vi "FGPA_HoppingStep(Nonlinear-ZOnly).vi"() -> ()   [LabVIEW 2014]
uses:
  <vilib>/Platform/TimedLoop/XDataNode/timing_clust.ctl
  <vilib>/Platform/TimedLoop/XDataNode/nitl_modes.ctl
  <vilib>/Platform/TimedLoop/XDataNode/wakeup.ctl
  <vilib>/rvi/Emulation/niFpgaSctlEmulationGetInTimedLoop.vi
  <vilib>/rvi/eio/common/nirviEmuTemplateMethod_errors.vi
  <vilib>/rvi/Emulation/niFpgaGetClockAttributes.vi
  <vilib>/rvi/Emulation/niFpgaEmulationReportErrorSimple.vi
  <vilib>/rvi/Emulation/niFpgaProcessEmulError.vi
  <vilib>/rvi/Emulation/niFpgaCriticalErrorInLSC.vi
  <vilib>/rvi/interface/RandomDataEmulation/niFpgaRandomDataHandleErrors.vi
  <vilib>/eio/EIONode/EIONode.xnode
  <vilib>/Platform/TimedLoop/XDataNode/XDataNode.xnode
  <vilib>/rvi/DataTransferAndStorage/Container/XNode/niFpgaContainer.xnode
  <vilib>/rvi/interface/RandomDataEmulation/nirviRandomDataFpgaReadWriteTemplate.vi
  <vilib>/Platform/TimedLoop/XDataNode/XDNodeRunTimeDep.lvlib
panel:
  in  "Relative?":bool
  in  "RelativeWithdraw":i16
  in  "BottomSleep us":i16=120
  in  "UpperSleep us":i16=120
  out "ZRealPos":i16
  out "Waveform Chart":i32(graph)
  in  "stop":bool
  out "Z":i32(graph)
  in  "ZOffset":i16
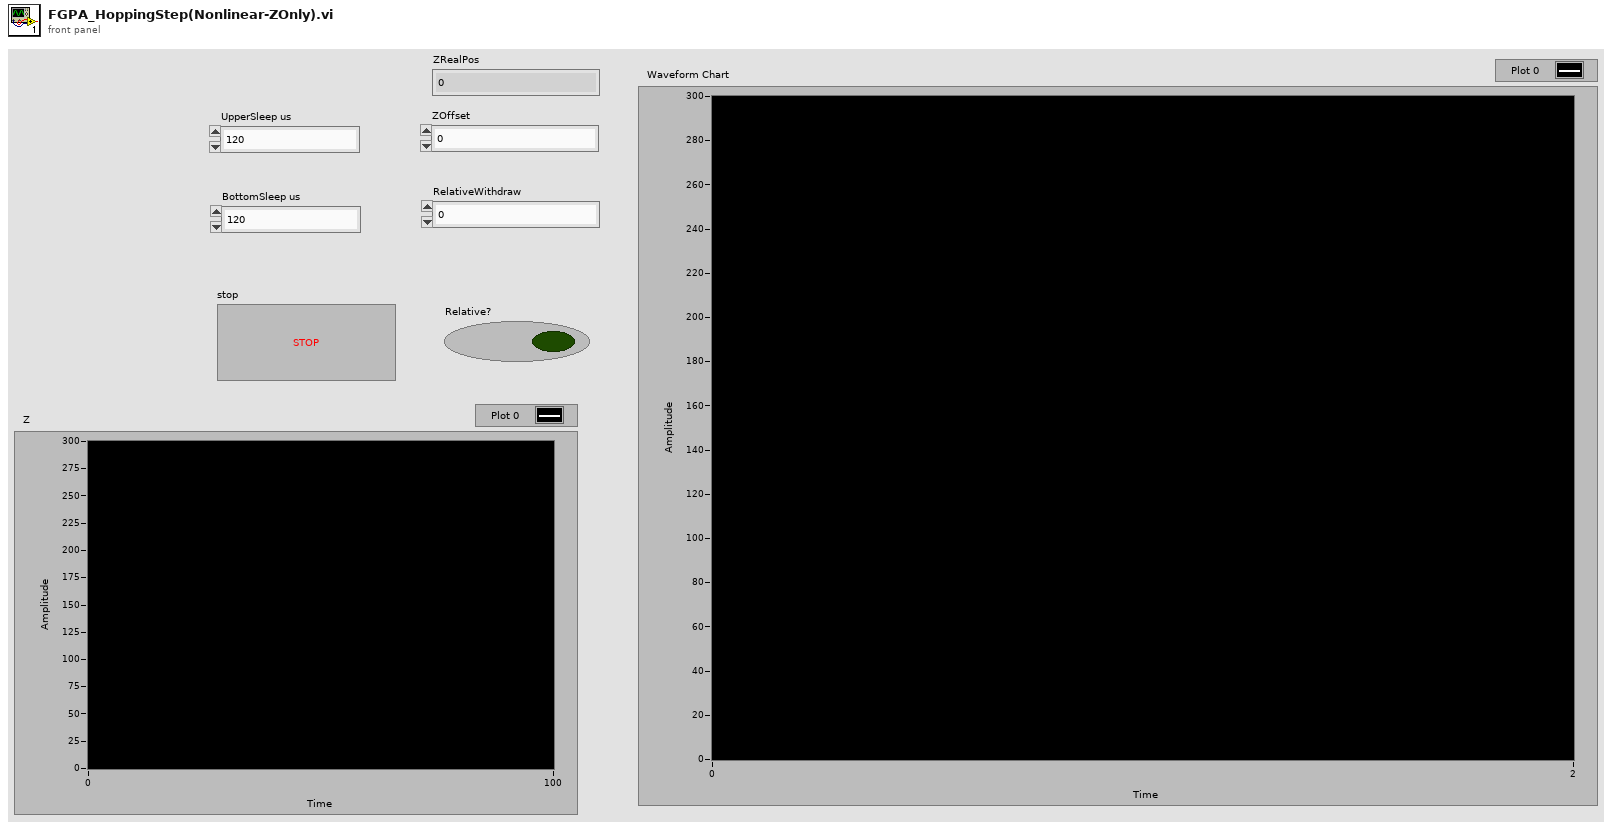
[diagram p1: front panel]
types:
  T1 = typedef "XDNodeRunTimeDep.lvlib/timing_clust.ctl" = cluster{"Expected End [f-1]":u64, "Actual End [f-1]":u64, "Finished Late? [f-1]":bool, "Expected End [i-1]":u64, "Actual End [i-1]":u64, "Finished Late? [i-1]":bool, "Expected Start [i]":u64, "Actual Start [i]":u64, "Expected Start [f]":u64, "Actual Start [f]":u64, "Source Name":string, "Structure Name":string, "Period":i64, "Deadline":i64, "Offset":i64, "Start":i64, "Priority":i32, "Timeout":i32, "Mode":T2, "Wakeup Reason":T3, "Error":errorcluster, "Source Type":string, "Secondary Source Type":string, "Global End Time":u64, "Global Start Time":u64, "Frame Duration":u64, "Iteration Duration":u64, "Assigned CPU":i32, "I/O Scan Engine Mode":u32}
  T2 = typedef "XDNodeRunTimeDep.lvlib/nitl_modes.ctl" = enum32{"No Change", "Process missed periods, maintain original phase", "Discard missed periods, maintain original phase", "Process missed periods, ignore original phase", "Discard missed periods, ignore original phase"}
  T3 = typedef "XDNodeRunTimeDep.lvlib/wakeup.ctl" = enum32{"Normal", "Aborted", "Asynchronous wakeup", "Timing source error", "Timed loop error", "Timeout"}
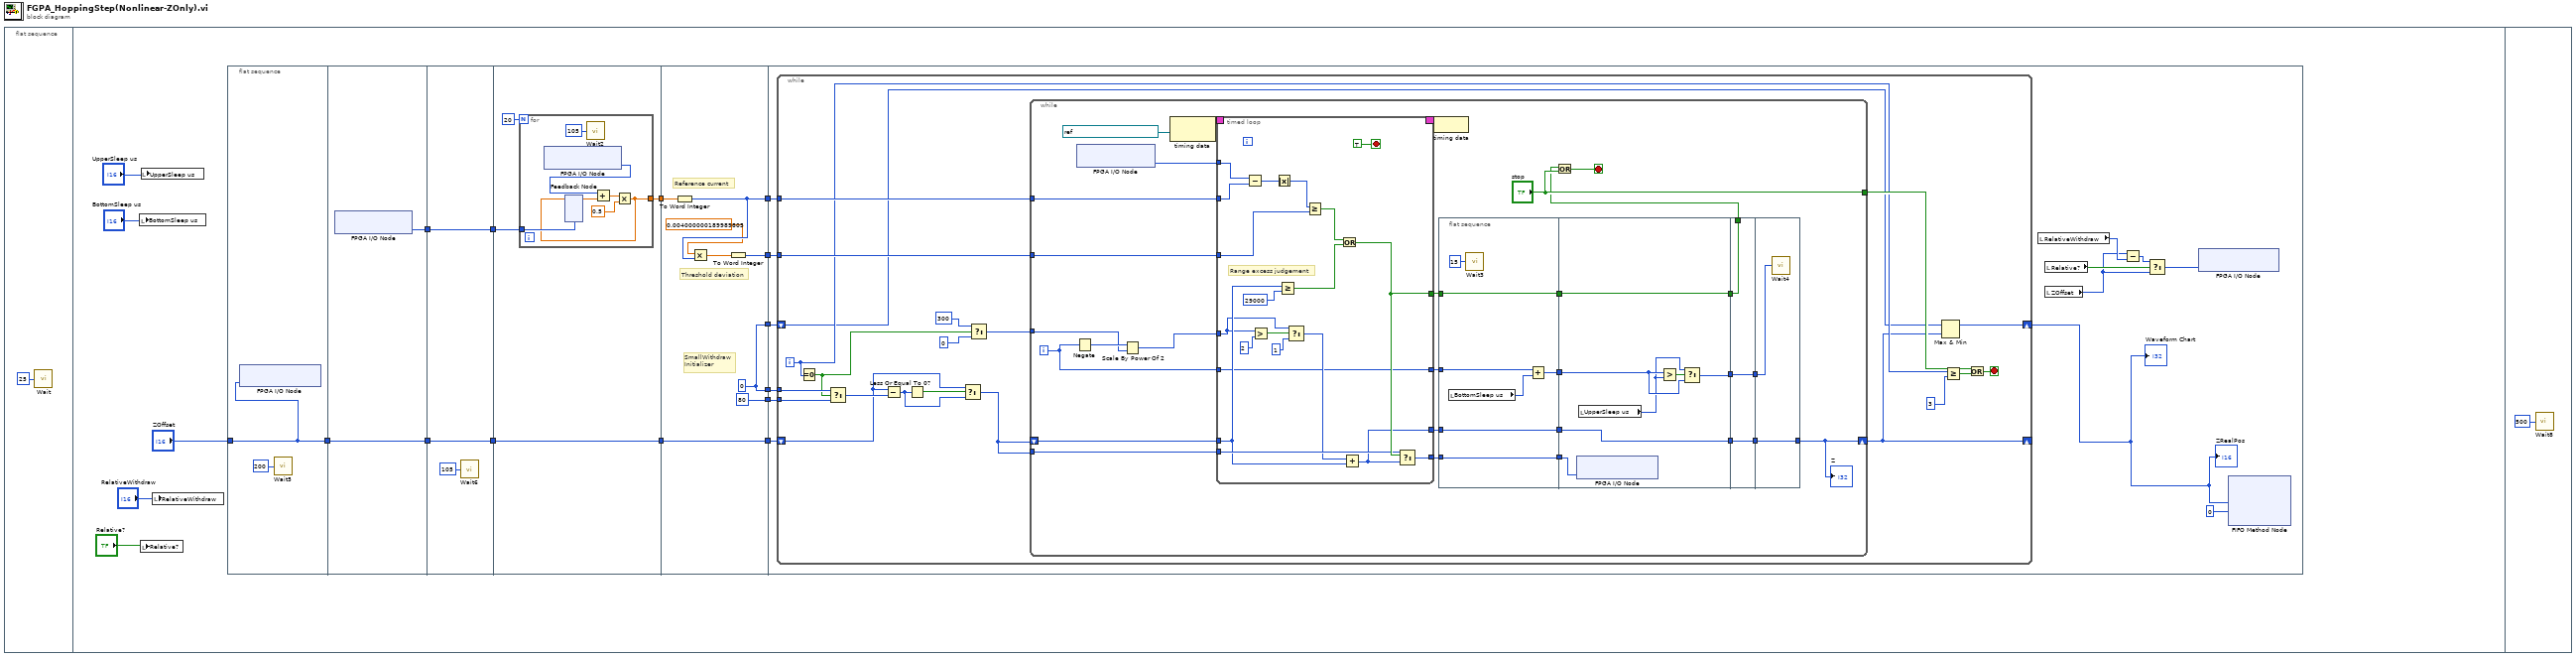
[diagram p0: block diagram]
diagram:
  n1 = flat-sequence {
    frame #0 {
      n2 = call "Wait"("Count(mSec)"=u32 25 ("Count(uSec)")) -> ()  [unwired: 1 out]
    }
    frame #1 {
      n3 = local write "BottomSleep us"("BottomSleep us") -> ()
      n4 = local write "Relative?"("Relative?") -> ()
      n5 = local write "UpperSleep us"("UpperSleep us") -> ()
      n6 = local write "RelativeWithdraw"("RelativeWithdraw") -> ()
      n7 = flat-sequence {
        tunnel: [w20] -> w10
        tunnel: "ZOffset" -> [w20]
        tunnel: [w22] -> w9
        tunnel: w10 -> [w23]
        tunnel: [w23] -> w7
        tunnel: w9 -> [w26]
        tunnel: [w26] -> w8
        tunnel: w7 -> [w25]
        tunnel: [w25] -> w6
        tunnel: w8 -> [w30]
        tunnel: [w28] -> w18
        tunnel: [w27] -> w17
        tunnel: w6 -> [w27]
        tunnel: [w39] -> w14
        tunnel: w18 -> [w45]
        tunnel: [w44] -> w15
        tunnel: [w41] -> w16
        tunnel: [i16 80] -> w13
        tunnel: w17 -> [w39]
        tunnel: [w38] -> w12
        tunnel: [w38] -> w11
        tunnel: w16 -> [w56]
        tunnel: w15 -> [w57]
        tunnel: w14 -> [w58]
        tunnel: w13 -> [w55]
        tunnel: w12 -> [w54]
        tunnel: w11 -> [w53]
        frame #0 {
          n8 = xnode "FPGA I/O Node"("Connector0/AO0"=w20) -> ()  [unwired: 1 in, 1 out]
          n9 = call "Wait5"("Count(uSec)"=u32 200) -> ()  [unwired: 1 out]
        }
        frame #1 {
          n10 = xnode "FPGA I/O Node"() -> ("Connector0/AI1"=w22:i16)  [unwired: 1 in, 1 out]
        }
        frame #2 {
          n11 = call "Wait6"("Count(uSec)"=u32 105) -> ()  [unwired: 1 out]
        }
        frame #3 {
          n12 = for {
            N: 20 -> [_]
            tunnel: w30 -> [w36]
            tunnel: [w31] -> w28
            n13 = xnode "FPGA I/O Node"() -> ("Connector0/AI1"=w34:i16)  [unwired: 1 in, 1 out]
            n14 = feedback #1(w36) -> (w35:sgl)
            n15 = call "Wait2"("Count(uSec)"=u32 105) -> ()  [unwired: 1 out]
            n16 = Add(x=w34, y=w35) -> (x+y=w33:sgl)
            n17 = Multiply(x=w33, y=sgl 0.5) -> (x*y=w31:sgl)
            n18 = feedback-in #1(w31) -> ()
          }
        }
        frame #4 {
          w38 = i16 0
          # "SmallWithdraw\nInitializer"
          # "Threshold deviation"
          # "Reference current"
          n19 = To Word Integer(number=w45) -> (16bit integer=w44:i16)
          n20 = Multiply(x=sgl 0.004, y=w44) -> (x*y=w42:sgl)
          n21 = To Word Integer(number=w42) -> (16bit integer=w41:i16)
        }
        frame #5 {
          n22 = while {
            tunnel: w57 -> [w79]
            tunnel: w56 -> [w78]
            tunnel: w55 -> [w73]
            shift-right: [w65] -> _
            shift-left: w58 -> [w70]
            tunnel: w54 -> [w67]
            shift-right: [w64] -> w46
            shift-left: w53 -> [w66]
            i -> [w74]
            stop <- w77 stop-if-true
            n23 = Equal To 0?(x=w74) -> (x = 0?=w63:bool)
            n24 = Select(t=w67, s=w63, f=w73) -> (s? t:f=w72:i16)
            n25 = Subtract(x=w70, y=w72) -> (x-y=w69:i32)
            n26 = Less Or Equal To 0?(x=w69) -> (x <= 0?=w71:bool)
            n27 = Select(t=w70, s=w71, f=w69) -> (s? t:f=w68:i32)
            n28 = Select(t=i16 300, s=w63, f=i16 0) -> (s? t:f=w60:i16)
            n29 = while {
              tunnel: w79 -> [w101]
              tunnel: w78 -> [w103]
              tunnel: ["stop"] -> w75
              shift-right: [w92] -> w65
              shift-left: w68 -> [w98]
              tunnel: w68 -> [w95]
              tunnel: w60 -> [w82]
              i -> [w80]
              stop <- w105 stop-if-true
              n30 = Negate(x=w80) -> (-x=w83:i32)
              n31 = xnode "FPGA I/O Node"() -> ("Connector0/AI1"=w102:i16)  [unwired: 1 in, 1 out]
              n32 = Scale By Power Of 2(n=w83, x=w82) -> (x*2^n=w81:i16)
              n33 = node-c288(refnum<k21> "40 MHz Onboard Clock" ("Source Name")) -> (w108:T1)
              n34 = timed-loop {
                timing: w108 -> [_]
                timing-out: [_] -> w107
                tunnel: w101 -> [w145]
                tunnel: w103 -> [w128]
                tunnel: w102 -> [w146]
                tunnel: [w141] -> w99
                tunnel: [w140] -> w97
                tunnel: w98 -> [w137]
                tunnel: w95 -> [w139]
                tunnel: [w136] -> w94
                tunnel: w81 -> [w131]
                tunnel: [w133] -> w84
                tunnel: w80 -> [w133]
                stop <- TRUE stop-if-true
                # "Range excess judgement"
                n35 = Subtract(x=w146, y=w145) -> (x-y=w129:i16)
                n36 = Greater?(x=w131, y=i16 2) -> (0:w130:bool)
                n37 = Absolute Value(x=w129) -> (abs(x)=w144:i16)
                n38 = Greater Or Equal?(x=w137, y=i16 29000) -> (x >= y?=w142:bool)
                n39 = Select(t=w131, s=w130, f=1) -> (s? t:f=w134:i32)
                n40 = Greater Or Equal?(x=w144, y=w128) -> (x >= y?=w143:bool)
                n41 = Or(x=w143, y=w142) -> (x .or. y?=w140:bool)
                n42 = Add(x=w134, y=w137) -> (x+y=w136:i32)
                n43 = Select(t=w139, s=w140, f=w136) -> (s? t:f=w141:i32)
              }
              n44 = node-c288(w107) -> ()
              n45 = flat-sequence {
                tunnel: [w114] -> w100
                tunnel: w99 -> [w114]
                tunnel: w97 -> [w113]
                tunnel: [w113] -> w96
                tunnel: w94 -> [w112]
                tunnel: [w112] -> w93
                tunnel: [w110] -> w85
                tunnel: w84 -> [w111]
                tunnel: w100 -> [w120]
                tunnel: [w122] -> w91
                tunnel: w96 -> [w121]
                tunnel: w93 -> [w122]
                tunnel: [w121] -> w89
                tunnel: [w118] -> w86
                tunnel: w85 -> [w117]
                tunnel: w91 -> [w125]
                tunnel: [w125] -> w90
                tunnel: w89 -> [w124]
                tunnel: [w124] -> w88
                tunnel: [w123] -> w87
                tunnel: w86 -> [w123]
                tunnel: w90 -> [w127]
                tunnel: [w127] -> w92
                tunnel: w87 -> [w126]
                frame #0 {
                  n46 = local read "BottomSleep us"() -> (w109:i16)
                  n47 = call "Wait3"("Count(uSec)"=u32 15) -> ()  [unwired: 1 out]
                  n48 = Add(x=w111, y=w109) -> (x+y=w110:i32)
                }
                frame #1 {
                  n49 = xnode "FPGA I/O Node"("Connector0/AO0"=w120) -> ()  [unwired: 1 in, 1 out]
                  n50 = local read "UpperSleep us"() -> (w116:i16)
                  n51 = Greater?(x=w117, y=w116) -> (0:w119:bool)
                  n52 = Select(t=w116, s=w119, f=w117) -> (s? t:f=w118:i32)
                }
                frame #2 {
                }
                frame #3 {
                  n53 = call "Wait4"("Count(uSec)"=w126) -> ()  [unwired: 1 out]
                }
              }
              n54 = Or(x=w88, y="stop") -> (x .or. y?=w105:bool)
              "Z" <- w92
            }
            n55 = Max & Min(x=w66, y=w65) -> (max(x,y)=w64:i32)  [unwired: 1 out]
            n56 = Greater Or Equal?(x=w74, y=3) -> (x >= y?=w76:bool)
            n57 = Or(x=w75, y=w76) -> (x .or. y?=w77:bool)
          }
          "Waveform Chart" <- w46
          "ZRealPos" <- w46
          n58 = local read "RelativeWithdraw"() -> (w50:i16)
          n59 = local read "Relative?"() -> (w52:bool)
          n60 = local read "ZOffset"() -> (w49:i16)
          n61 = Subtract(x=w49, y=w50) -> (x-y=w51:i16)
          n62 = Select(t=w51, s=w52, f=w49) -> (s? t:f=w48:i16)
          n63 = xnode "FPGA I/O Node"("Connector0/AO0"=w48) -> ()  [unwired: 1 in, 1 out]
          n64 = xnode ("FIFO Method Node")("Element"=w46, "Timeout"=0) -> ()  [unwired: 1 in, 2 out]
        }
      }
    }
    frame #2 {
      n65 = call "Wait8"("Count(uSec)"=u32 500) -> ()  [unwired: 1 out]
    }
  }
